vi "Core Action.vi"(8 "error in (no error)":errorcluster, 10 "SECS-II Class":refnum<class "SECS-II Class.lvclass">, 11 "Host Requests Status Equipment Constant Namelist in":refnum<class "06-Host Requests Status Equipment Constant Namelist.lvclass">) -> (0 "error out":errorcluster, 2 "SECS-II Class Out":refnum<class "SECS-II Class.lvclass">, 3 "Host Requests Status Equipment Constant Namelist out":refnum<class "06-Host Requests Status Equipment Constant Namelist.lvclass">)   [LabVIEW 2020, in "SECS Scenarios.lvlib" / "06-Host Requests Status Equipment Constant Namelist.lvclass"]
uses:
  06-Host Requests Status Equipment Constant Namelist.lvclass
  D:/Dropbox/SECS/SECS_GEM v1.1.0/Com/SECS Scenarios/Scenarios Class/Scenarios Class.lvclass
  SECS Communication/SECS-II Class/SECS-II Class.lvclass
  SECS Communication/S2 Message Class/S2 Message Class.lvclass
  D:/Dropbox/SECS/SECS_GEM v1.1.0/Com/SECS Communication/SECS-II Class/SECS-II Class.lvclass
  Scenarios Class/Reply State.ctl
  Scenarios Class/Scenarios Class.lvclass/Scenarios Class.ctl
  Scenarios Class/Write Reply State.vi
  Scenarios Class/Read HSMS Class.vi
  SECS Communication/SECS Data Class/Get ECID Data.vi
  SECS Communication/SECS Data Class/Get All ECID Data.vi
  SECS Communication/HSMS Class/HSMS Class.lvclass
  SECS Communication/SECS Data Class/SECS Data Class.lvclass
  Scenarios Class/Scenarios Class.lvclass
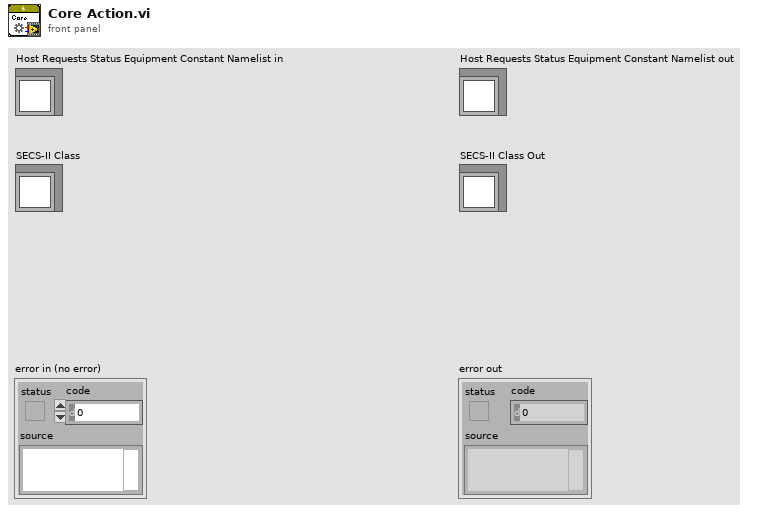
[diagram p1: front panel]
types:
  T1 = typedef "SECS Scenarios.lvlib/Scenarios Class.lvclass/Reply State.ctl" = enum16{"OK", "Illegal Data", "Unknown Stream", "Unknown Function", "Off-Line", "T3 Timeout", "Inner-Timeout"}
  T2 = cluster{"ECID":u32, "ECNAME":string, "ECMIN":string, "ECMAX":string, "ECDEF":string, "UNITS":string}
  T3 = typedef "SECS Communication.lvlib/SECS Data Class.lvclass/ECID Data.ctl" = cluster{"ECID":u32, "Name":string, "Description":string, "Format Code":T4, "Unit":string, "Max":dbl, "Min":dbl, "Default":string, "Source":string, "Data":variant}
  T4 = typedef "SECS Communication.lvlib/SECS-II Class.lvclass/Format Code.ctl" = enum16{"L", "A", "B", "Boolean", "J", "I1", "I2", "I4", "I8", "U1", "U2", "U4", "U8", "F4", "F8", "Char"}
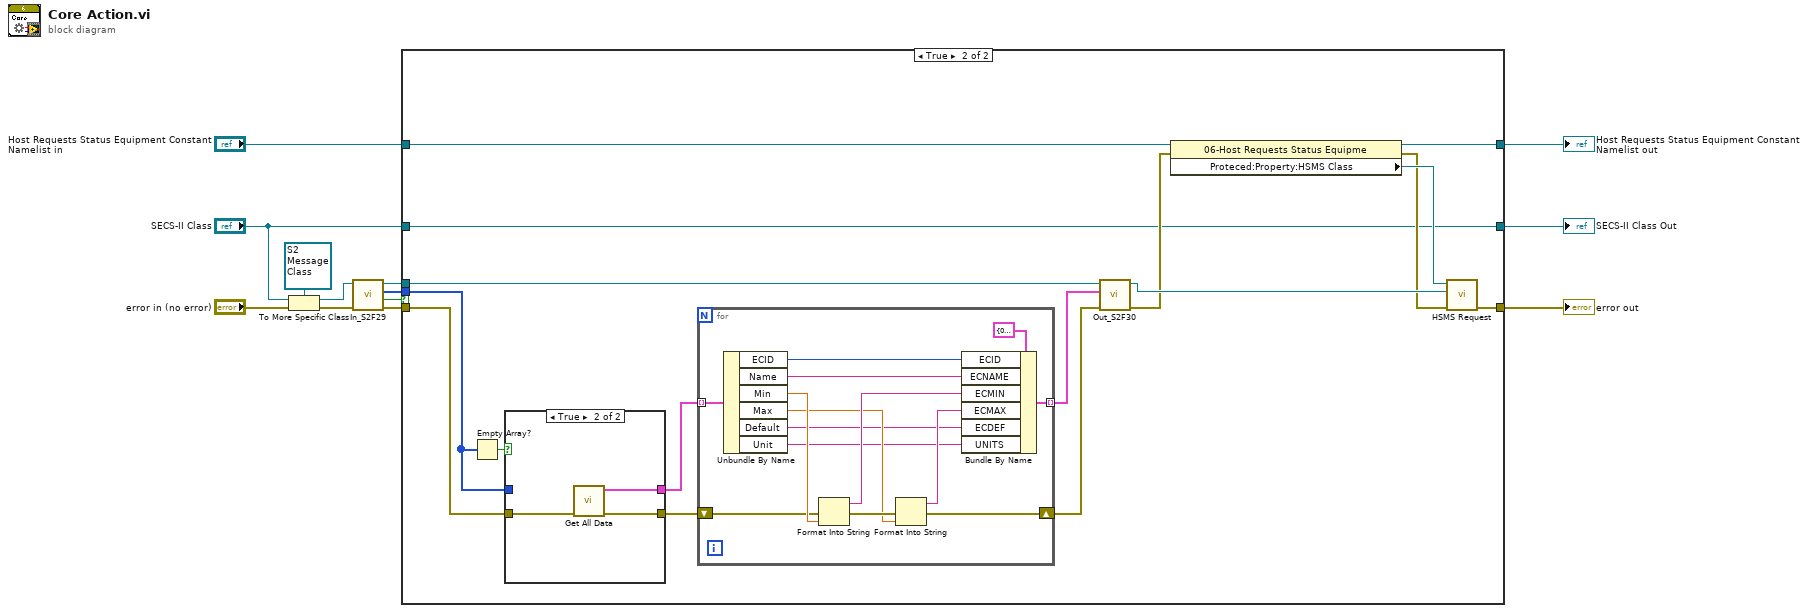
[diagram p0: block diagram]
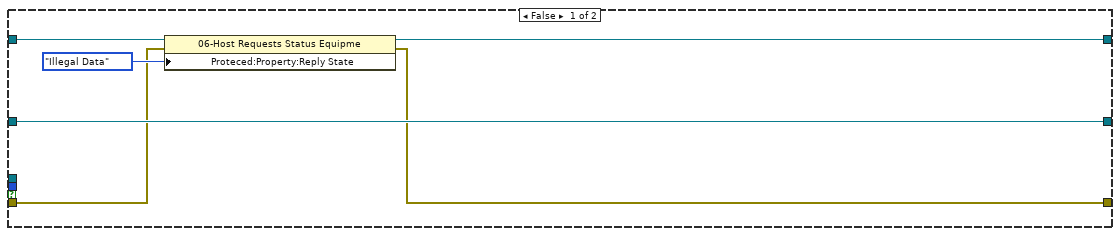
[diagram p2: hidden frame]
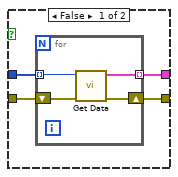
[diagram p3: hidden frame]
diagram:
  n1 = To More Specific Class(target class=refnum<class "S2 Message Class.lvclass"> refnum ("SECS Communication.lvlib:S2 Message Class.lvclass"), reference="SECS-II Class", error in="error in (no error)") -> (specific class reference=w10:refnum<class "S2 Message Class.lvclass">, error out=w11:errorcluster)
  n2 = call "In_S2F29.vi"("error in (no error)"=w11, "S2 Message Class in"=w10) -> ("error out"=w6:errorcluster, "OK?"=w3:bool, "Equipment Constant ID(ECID)"=w5:u32[], "S2 Message Class out"=w9:refnum<class "S2 Message Class.lvclass">)  [unwired: 6 in]
  n3 = case shown="True" w3 {
    tunnel: "Host Requests Status Equipment Constant Namelist in" -> [w18 w34]
    tunnel: w9 -> [_ w33]
    tunnel: [w14 w29] -> w8
    tunnel: [w15 w28] -> w7
    tunnel: w6 -> [w16 w26]
    tunnel: w5 -> [_ w25]
    tunnel: "SECS-II Class" -> [w19 w20]
    tunnel: [w19 w20] -> w1
    frame False {
      n4 = property class="06-Host Requests Status Equipme"(reference=w18, error in=w16, "Proteced:Property:Reply State"=Reply_State."Illegal Data" ("Reply State")) -> (reference out=w15:refnum<class "06-Host Requests Status Equipment Constant Namelist.lvclass">, error out=w14:errorcluster)
    }
    frame True {
      n5 = Empty Array?(array=w25) -> (empty?=w24:bool)
      n6 = case shown="True" w24 {
        tunnel: [w39 w44] -> w27
        tunnel: w26 -> [w38 w46]
        tunnel: w25 -> [w37 _]
        tunnel: [w36 w45] -> w23
        frame False {
          n7 = for {
            shift-right: [w43] -> w39
            shift-left: w38 -> [w42]
            tunnel: w37 -> [w41] mode=indexing
            tunnel: [w40] -> w36 mode=indexing
            n8 = call-poly "Get Data.vi"("error in"=w42, "ECID"=w41) -> ("error out"=w43:errorcluster, "ECID Data"=w40:T3)  [unwired: 7 in, 1 out]
          }
        }
        frame True {
          n9 = call-poly "Get All Data.vi"("error in (no error)"=w46) -> ("error out"=w44:errorcluster, "ECID Data"=w45:T3[])  [unwired: 9 in]
        }
      }
      n10 = for {
        shift-right: [w50] -> w31
        shift-left: w27 -> [w49]
        tunnel: [w59] -> w32 mode=indexing
        tunnel: w23 -> [w48] mode=indexing
        n11 = Unbundle By Name(w48) -> ("ECID"=w47:u32, "Name"=w60:string, "Min"=w57:dbl, "Max"=w54:dbl, "Default"=w52:string, "Unit"=w51:string)
        n12 = Format Into String(error in=w49, w57) -> (resulting string=w56:string, error out=w55:errorcluster)  [unwired: 2 in]
        n13 = Format Into String(error in=w55, w54) -> (resulting string=w53:string, error out=w50:errorcluster)  [unwired: 2 in]
        n14 = Bundle By Name(cluster=T2 {"ECID"=0, "ECNAME"="", "ECMIN"="", "ECMAX"="", "ECDEF"="", "UNITS"=""} ("S2F30"), "ECID"=w47, "ECNAME"=w60, "ECMIN"=w56, "ECMAX"=w53, "ECDEF"=w52, "UNITS"=w51) -> (w59:T2)
      }
      n15 = call "Out_S2F30.vi"("error in (no error)"=w31, "S2F30"=w32, "S2 Message Class in"=w33) -> ("error out"=w22:errorcluster, "S2 Message Class out"=w30:refnum<class "S2 Message Class.lvclass">)  [unwired: 7 in]
      n16 = property class="06-Host Requests Status Equipme"(reference=w34, error in=w22) -> (reference out=w28:refnum<class "06-Host Requests Status Equipment Constant Namelist.lvclass">, error out=w21:errorcluster, "Proteced:Property:HSMS Class"=w35:refnum<class "HSMS Class.lvclass">)
      n17 = call "HSMS Request.vi"("error in (no error)"=w21, "SECS-II Class In"=w30, "HSMS Class in"=w35) -> ("error out"=w29:errorcluster)  [unwired: 7 in, 1 out]
    }
  }
  "error out" <- w8
  "Host Requests Status Equipment Constant Namelist out" <- w7
  "SECS-II Class Out" <- w1
